vi "Max To Normal.vi"(8 "error in (no error)":errorcluster, 10 "MouseCoords":cluster{"Horizontal":i32, "Vertical":i32}, 11 "MainUI in":refnum<class "UI_Top_Customer.lvclass">) -> (0 "error out":errorcluster, 3 "MainUI out":refnum<class "UI_Top_Customer.lvclass">)   [LabVIEW 2021, in "UI_Top_Customer.lvclass"]
uses:
  UI_Top_Customer.lvclass
  UI_Top_Customer.lvclass/UI_Top_Customer.ctl
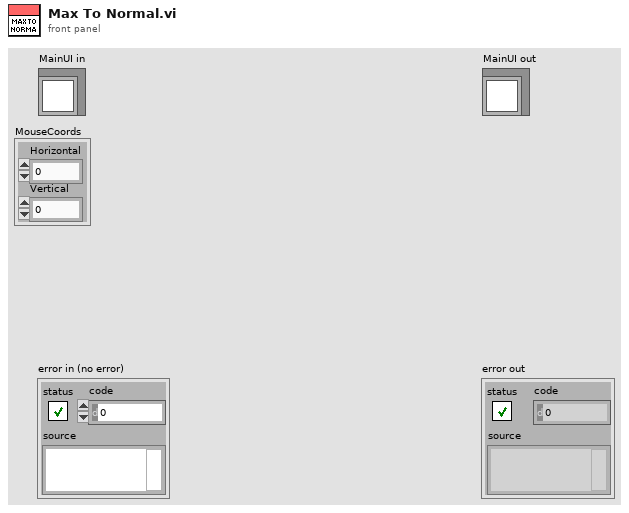
[diagram p1: front panel]
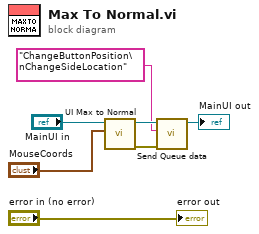
[diagram p0: block diagram]
diagram:
  n1 = call "UI Max to Normal.vi"("Coords"="MouseCoords", "MainUI in"="MainUI in") -> ("error out"=w3:errorcluster, "MainUI out"=w4:refnum<class "UI_Top_Customer.lvclass">)  [unwired: 8 in]
  n2 = call "Send Queue data.vi"("error in (no error)"=w3, "Elements at Back"="ChangeButtonPosition\nChangeSideLocation", "UI_Top_Customer in"=w4) -> ("UI_Top_Customer out"=→"MainUI out":refnum<class "UI_Top_Customer.lvclass">)  [unwired: 7 in, 1 out]
  "error out" <- "error in (no error)"
